vi "Run Step.vi"(0 "CAN Cmd Ref":refnum<vi>, 2 "FPGA Ref":T2, 3 "Stagger Time (ms)":i32, 4 "Cycles Completed in":u32, 5 "PWM Freq (Hz)":dbl, 7 "Controller Type:":T3, 8 "# of Steps":i32, 9 "Restarts Cluster":T4={"CMD Starts:"=[0, 0, 0, 0, 0, 0], "Restarts:"=[0, 0, 0, 0, 0, 0], "Total CMD:"=[0, 0, 0, 0, 0, 0], "Total Restarts:"=[0, 0, 0, 0, 0, 0]}, 10 "VoltCtrlRef":string, 13 "Stagger Counter":i32, 14 "Current Step in":i32, 15 "Last CMDs":dbl[](array[numeric]), 16 "Profile":string[][](array[string]), 17 "Pumps Present":u32) -> (12 "PS Cmd":dbl, 19 "Ignition Relays":T1, 20 "Manual CMDs":dbl[](array[numeric]), 21 "Current Step out":i32, 23 "Press Cmd":dbl, 24 "Cycles Completed out":u32, 25 "Step Time":dbl, 26 "Power Relays":T1, 27 "Restarts Cluster OUT":T4)   [LabVIEW 2013]
uses:
  Type Defs/Restarts Cluster.ctl
  Type Defs/Controller Names.ctl
  Controls/FPGA_Reference.ctl
  <vilib>/Utility/error.llb/Error Cluster From Error Code.vi
  <vilib>/rvi/errors/niLvFpgaAdjustHostInterfaceError.vi
  <vilib>/rvi/interface/nirviReadWriteControl/nirviReadWriteControl.xnode
  FPGA/bitfiles/TI sbRIO PWM (FPGA) v1.0.lvbitx
  NiFpgaLv.dll
  <vilib>/rvi/errors/niLvFpgaMergeErrorWithErrorCode.vi
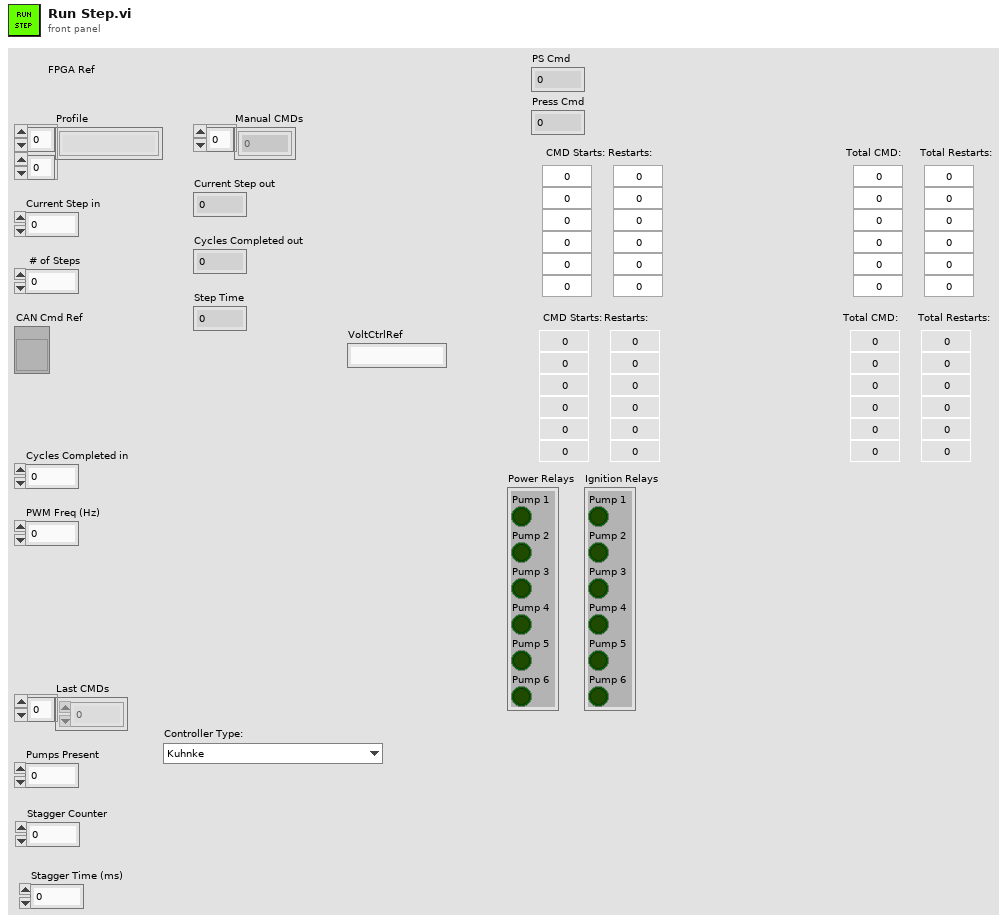
[diagram p1: front panel]
types:
  T1 = cluster{"Pump 1":bool, "Pump 2":bool, "Pump 3":bool, "Pump 4":bool, "Pump 5":bool, "Pump 6":bool}
  T2 = typedef "FPGA_Reference.ctl" = refnum<k20>
  T3 = typedef "Controller Names.ctl" = enum16{"Kuhnke", "Conti", "Helbako", "TI PWM", "PSA", "Hella Gas", "Hella Diesel", "8 Comm", "10 Comm", "8 Comm Hella", "10 Comm Hella", "8 Comm Omron", "10 Comm Omron", "8 Comm Nissan", "10 Comm Nissan"}
  T4 = typedef "Restarts Cluster.ctl" = cluster{"CMD Starts:":i32[], "Restarts:":i32[], "Total CMD:":i32[], "Total Restarts:":i32[]}
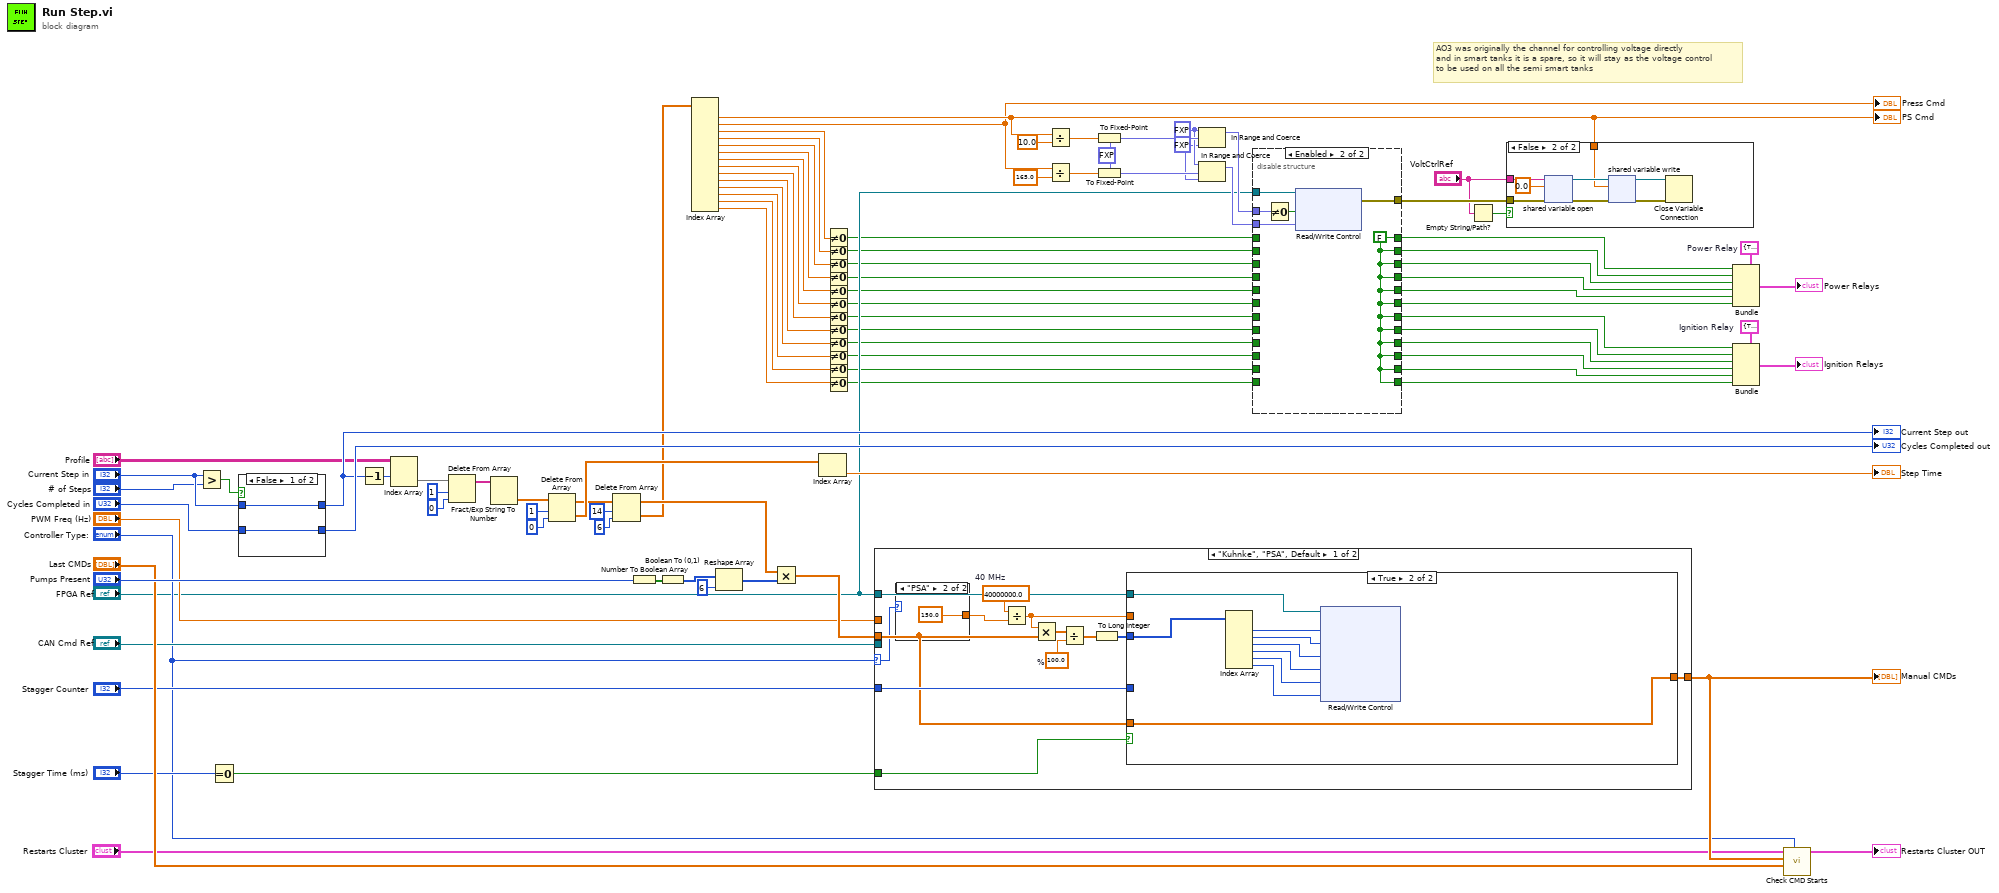
[diagram p0: block diagram]
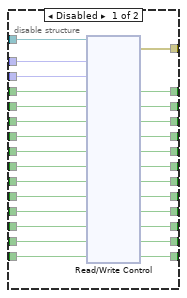
[diagram p2: hidden frame]
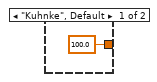
[diagram p4: hidden frame]
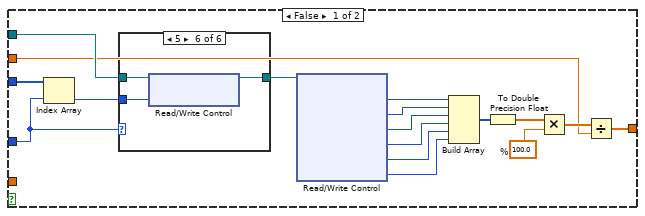
[diagram p5: hidden frame]
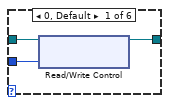
[diagram p6: hidden frame]
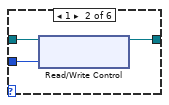
[diagram p7: hidden frame]
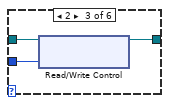
[diagram p8: hidden frame]
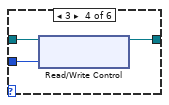
[diagram p9: hidden frame]
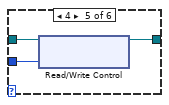
[diagram p10: hidden frame]
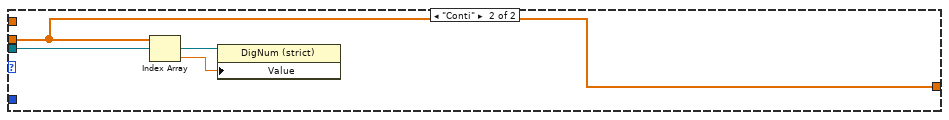
[diagram p11: hidden frame]
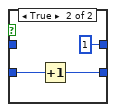
[diagram p12: hidden frame]
diagram:
  w30 = T1 {"Pump 1"=TRUE, "Pump 2"=TRUE, "Pump 3"=TRUE, "Pump 4"=TRUE, "Pump 5"=TRUE, "Pump 6"=TRUE}  # Ignition Relay
  w31 = T1 {"Pump 1"=TRUE, "Pump 2"=TRUE, "Pump 3"=TRUE, "Pump 4"=TRUE, "Pump 5"=TRUE, "Pump 6"=TRUE}  # Power Relay
  w50 = fxp<+/-,20,5> 0.0 ("lower limit")
  w51 = fxp<+/-,20,5> 5.0 ("upper limit")
  w63 = fxp<+/-,20,5> 0.0 ("AO0")
  # "AO3 was originally the channel for controlling voltage directly\nand in smart tanks it is a spare, so it will stay as the voltage control\nto be used on all the semi smart tanks"
  n1 = Greater?(x="Current Step in", y="# of Steps") -> (0:w88:bool)
  n2 = Equal To 0?(x="Stagger Time (ms)") -> (x = 0?=w66:bool)
  n3 = case shown="False" w88 {
    tunnel: [w97 1 ("Current Step")] -> w90
    tunnel: "Current Step in" -> [w97 _]
    tunnel: "Cycles Completed in" -> [w96 w99]
    tunnel: [w96 w98] -> w92
    frame False {
    }
    frame True {
      n4 = Increment(x=w99) -> (x+1=w98:u32)
    }
  }
  "Cycles Completed out" <- w92
  "Current Step out" <- w90
  n5 = Decrement(x=w90) -> (x-1=w76:i32)
  n6 = Index Array(array="Profile", index (row)=w76) -> (element=w77:string[])  [unwired: 1 in]
  n7 = Delete From Array(array=w77, length=1, index=0 ("length")) -> (array with subset deleted=w81:string[])  [unwired: 1 out]
  n8 = Fract/Exp String To Number(string=w81) -> (number=w84:dbl[])  [unwired: 3 in, 1 out]
  n9 = Delete From Array(array=w84, length=1, index=0 ("length")) -> (deleted portion=w85:dbl[], array with subset deleted=w73:dbl[])
  n10 = Delete From Array(array=w73, length=14, index=6) -> (deleted portion=w61:dbl[], array with subset deleted=w70:dbl[])
  n11 = Number To Boolean Array(number="Pumps Present") -> (Boolean array=w62:bool[])
  n12 = Boolean To (0,1)(Boolean=w62) -> (0, 1=w27:i16[])
  n13 = Index Array(array=w61) -> (element #1=w44:dbl, element #2=w43:dbl, element #3=w60:dbl, element #4=w42:dbl, element #5=w40:dbl, element #6=w41:dbl, element #7=w39:dbl, element #8=w38:dbl, element #9=w37:dbl, element #10=w35:dbl, element #11=w36:dbl, element #12=w34:dbl, element #13=w33:dbl, element #14=w32:dbl)  [unwired: 14 in]
  "PS Cmd" <- w44
  "Press Cmd" <- w43
  n14 = Reshape Array(w27, 6 ("dimension size")) -> (w26:i16[])
  n15 = Multiply(x=w70, y=w26) -> (x*y=w95:dbl[])
  n16 = Index Array(array=w85) -> (element=→"Step Time":dbl)  [unwired: 1 in]
  n17 = Not Equal To 0?(x=w60) -> (x != 0?=w24:bool)
  n18 = Not Equal To 0?(x=w42) -> (x != 0?=w23:bool)
  n19 = Not Equal To 0?(x=w40) -> (x != 0?=w22:bool)
  n20 = Not Equal To 0?(x=w41) -> (x != 0?=w21:bool)
  n21 = Not Equal To 0?(x=w39) -> (x != 0?=w20:bool)
  n22 = Not Equal To 0?(x=w38) -> (x != 0?=w19:bool)
  n23 = Not Equal To 0?(x=w37) -> (x != 0?=w18:bool)
  n24 = Not Equal To 0?(x=w35) -> (x != 0?=w17:bool)
  n25 = Not Equal To 0?(x=w36) -> (x != 0?=w16:bool)
  n26 = Not Equal To 0?(x=w34) -> (x != 0?=w15:bool)
  n27 = Not Equal To 0?(x=w33) -> (x != 0?=w14:bool)
  n28 = Not Equal To 0?(x=w32) -> (x != 0?=w13:bool)
  n29 = case shown="\"Kuhnke\", \"PSA\", Default" "Controller Type:" {
    selector: "Controller Type:" -> [w102 _]
    tunnel: "PWM Freq (Hz)" -> [_ _]
    tunnel: w95 -> [w103 w160]
    tunnel: "FPGA Ref" -> [w108 _]
    tunnel: "CAN Cmd Ref" -> [_ w161]
    tunnel: "Stagger Counter" -> [w107 _]
    tunnel: [w105 w160] -> w68
    tunnel: w66 -> [w104 _]
    frame "Kuhnke", "PSA", Default {
      w112 = 40000000.0  # 40 MHz
      w110 = 100.0  # %
      n30 = case shown="\"PSA\"" w102 {
        tunnel: [100.0 ("y") 150.0 ("y")] -> w101
        frame "Kuhnke", Default {
        }
        frame "PSA" {
        }
      }
      n31 = Divide(x=w112, y=w101) -> (x/y=w106:dbl)
      n32 = Multiply(x=w106, y=w103) -> (x*y=w109:dbl[])
      n33 = Divide(x=w109, y=w110) -> (x/y=w111:dbl[])
      n34 = To Long Integer(number=w111) -> (32bit integer=w113:i32[])
      n35 = case shown="True" w104 {
        tunnel: w113 -> [w132 w159]
        tunnel: w108 -> [w131 w151]
        tunnel: w107 -> [w129 _]
        tunnel: w106 -> [w117 _]
        tunnel: [w116 w158] -> w105
        tunnel: w103 -> [_ w158]
        frame False {
          w119 = 100.0  # %
          n36 = Index Array(array=w132, index=w129) -> (element=w130:i32)
          n37 = case shown="5" w129 {
            tunnel: w131 -> [w135 w138 w141 w144 w147 w150]
            tunnel: w130 -> [w134 w137 w140 w143 w146 w149]
            tunnel: [w133 w136 w139 w142 w145 w148] -> w128
            frame 0, Default {
              n38 = xnode "Read/Write Control"("FPGA VI Reference In"=w135, "Duty (Ticks) 1"=w134) -> ("FPGA VI Reference Out"=w133:T2)  [unwired: 1 in, 1 out]
            }
            frame 1 {
              n39 = xnode "Read/Write Control"("FPGA VI Reference In"=w138, "Duty (Ticks) 2"=w137) -> ("FPGA VI Reference Out"=w136:T2)  [unwired: 1 in, 1 out]
            }
            frame 2 {
              n40 = xnode "Read/Write Control"("FPGA VI Reference In"=w141, "Duty (Ticks) 3"=w140) -> ("FPGA VI Reference Out"=w139:T2)  [unwired: 1 in, 1 out]
            }
            frame 3 {
              n41 = xnode "Read/Write Control"("FPGA VI Reference In"=w144, "Duty (Ticks) 4"=w143) -> ("FPGA VI Reference Out"=w142:T2)  [unwired: 1 in, 1 out]
            }
            frame 4 {
              n42 = xnode "Read/Write Control"("FPGA VI Reference In"=w147, "Duty (Ticks) 5"=w146) -> ("FPGA VI Reference Out"=w145:T2)  [unwired: 1 in, 1 out]
            }
            frame 5 {
              n43 = xnode "Read/Write Control"("FPGA VI Reference In"=w150, "Duty (Ticks) 6"=w149) -> ("FPGA VI Reference Out"=w148:T2)  [unwired: 1 in, 1 out]
            }
          }
          n44 = xnode "Read/Write Control"("FPGA VI Reference In"=w128) -> ("Duty (Ticks) 1"=w127:i32, "Duty (Ticks) 2"=w126:i32, "Duty (Ticks) 3"=w125:i32, "Duty (Ticks) 4"=w124:i32, "Duty (Ticks) 5"=w123:i32, "Duty (Ticks) 6"=w122:i32)  [unwired: 1 in, 2 out]
          n45 = Build Array(w127, w126, w125, w124, w123, w122) -> (w121:i32[])
          n46 = To Double Precision Float(number=w121) -> (double precision float=w120:dbl[])
          n47 = Multiply(x=w120, y=w119) -> (x*y=w118:dbl[])
          n48 = Divide(x=w118, y=w117) -> (x/y=w116:dbl[])
        }
        frame True {
          n49 = Index Array(array=w159) -> (element #1=w157:i32, element #2=w156:i32, element #3=w155:i32, element #4=w154:i32, element #5=w153:i32, element #6=w152:i32)  [unwired: 6 in]
          n50 = xnode "Read/Write Control"("FPGA VI Reference In"=w151, "Duty (Ticks) 1"=w157, "Duty (Ticks) 2"=w156, "Duty (Ticks) 3"=w155, "Duty (Ticks) 4"=w154, "Duty (Ticks) 5"=w153, "Duty (Ticks) 6"=w152) -> ()  [unwired: 1 in, 2 out]
        }
      }
    }
    frame "Conti" {
      n51 = Index Array(array=w160) -> (element=w162:dbl)  [unwired: 1 in]
      n52 = property class="DigNum (strict)"(reference=w161, "Value"=w162) -> ()  [unwired: 1 in, 2 out]
    }
  }
  "Manual CMDs" <- w68
  n53 = Divide(x=w44, y=10.0) -> (x/y=w54:dbl)
  n54 = Divide(x=w43, y=165.0) -> (x/y=w55:dbl)
  n55 = To Fixed-Point(fixed-point type=w63, number=w54) -> (fixed-point=w59:fxp<+/-,20,5>)
  n56 = To Fixed-Point(fixed-point type=w63, number=w55) -> (fixed-point=w58:fxp<+/-,20,5>)
  n57 = In Range and Coerce(upper limit=w51, x=w59, lower limit=w50) -> (coerced(x)=w52:fxp<+/-,20,5>)  [unwired: 1 out]
  n58 = In Range and Coerce(upper limit=w51, x=w58, lower limit=w50) -> (coerced(x)=w53:fxp<+/-,20,5>)  [unwired: 1 out]
  n59 = disable-structure shown="Enabled" {
    disable-tunnel: w53 -> [w178 w182]
    disable-tunnel: w52 -> [w177 w180]
    disable-tunnel: [w176 w183] -> w48
    disable-tunnel: "FPGA Ref" -> [w175 w184]
    disable-tunnel: w24 -> [w174 _]
    disable-tunnel: w23 -> [w173 _]
    disable-tunnel: w22 -> [w172 _]
    disable-tunnel: w21 -> [w171 _]
    disable-tunnel: w20 -> [w170 _]
    disable-tunnel: w19 -> [w169 _]
    disable-tunnel: w18 -> [w168 _]
    disable-tunnel: w17 -> [w167 _]
    disable-tunnel: w16 -> [w166 _]
    disable-tunnel: w14 -> [w164 _]
    disable-tunnel: w15 -> [w165 _]
    disable-tunnel: w13 -> [w163 _]
    disable-tunnel: [w174 w181] -> w12
    disable-tunnel: [w173 w181] -> w11
    disable-tunnel: [w172 w181] -> w10
    disable-tunnel: [w171 w181] -> w9
    disable-tunnel: [w170 w181] -> w8
    disable-tunnel: [w169 w181] -> w7
    disable-tunnel: [w168 w181] -> w6
    disable-tunnel: [w167 w181] -> w5
    disable-tunnel: [w166 w181] -> w4
    disable-tunnel: [w165 w181] -> w3
    disable-tunnel: [w164 w181] -> w2
    disable-tunnel: [w163 w181] -> w1
    frame Disabled {
      n60 = xnode "Read/Write Control"("FPGA VI Reference In"=w175, "AO3"=w177, "AO0"=w178, "DIO6"=w174, "DIO7"=w173, "DIO8"=w172, "DIO9"=w171, "DIO10"=w170, "DIO11"=w169, "DIO12"=w168, "DIO13"=w167, "DIO14"=w166, "DIO15"=w165, "DIO16"=w164, "DIO17"=w163) -> ("error out"=w176:errorcluster)  [unwired: 1 in, 1 out]
    }
    frame Enabled {
      w181 = FALSE
      n61 = Not Equal To 0?(x=w180) -> (x != 0?=w179:bool)
      n62 = xnode "Read/Write Control"("FPGA VI Reference In"=w184, "PS Control"=w179, "AO0"=w182) -> ("error out"=w183:errorcluster)  [unwired: 1 in, 1 out]
    }
  }
  n63 = Empty String/Path?(string/path="VoltCtrlRef") -> (empty?=w49:bool)
  n64 = case shown="False" w49 {
    tunnel: w48 -> [_ w188]
    tunnel: w44 -> [_ w186]
    tunnel: "VoltCtrlRef" -> [_ w185]
    frame True {
    }
    frame False {
      n65 = shared-variable-open(w185, w188, 0.0) -> (w192:refnum<k21>, w189:errorcluster)  [unwired: 1 in]
      n66 = shared-variable-write(w192, w189, w186) -> (w191:refnum<k21>, w190:errorcluster)
      n67 = Close Variable Connection(8:w190, 11:w191) -> ()  [unwired: 1 out]
    }
  }
  n68 = Bundle(cluster=w31, "Pump 1"=w12, "Pump 2"=w11, "Pump 3"=w10, "Pump 4"=w9, "Pump 5"=w8, "Pump 6"=w7) -> (→"Power Relays":T1)
  n69 = Bundle(cluster=w30, "Pump 1"=w6, "Pump 2"=w5, "Pump 3"=w4, "Pump 4"=w3, "Pump 5"=w2, "Pump 6"=w1) -> (→"Ignition Relays":T1)
  n70 = call "Check CMD Starts.vi"("Controller Type:"="Controller Type:", "Last CMDs"="Last CMDs", "Current CMDs"=w68, "Restarts Cluster IN"="Restarts Cluster") -> ("Restarts Cluster OUT"=→"Restarts Cluster OUT":T4)  [unwired: 7 in]
